vi "DSF.Engine.Memory.Cache.Plugin.Get Transfer Caches.vi"(8 "error in (no error)":errorcluster, 11 "Plugin Cache in":refnum<class "DSF.Engine.Memory.Cache.Plugin.lvclass">) -> (0 "error out":errorcluster, 2 "Transfer Caches":refnum<class "DSF.Engine.Memory.Cache.Transfer.lvclass">[](array[class]), 3 "Plugin Cache out":refnum<class "DSF.Engine.Memory.Cache.Plugin.lvclass">)   [LabVIEW 2016, in "DSF.Engine.lvlib" / "DSF.Engine.Memory.Cache.Plugin.lvclass"]
uses:
  DSF.Engine.Memory.Cache.Plugin.lvclass
  DSF.Engine.Memory.Cache.Transfer.lvclass
  DSF.Engine.Memory.Cache.Plugin.lvclass/DSF.Engine.Memory.Cache.Plugin.ctl
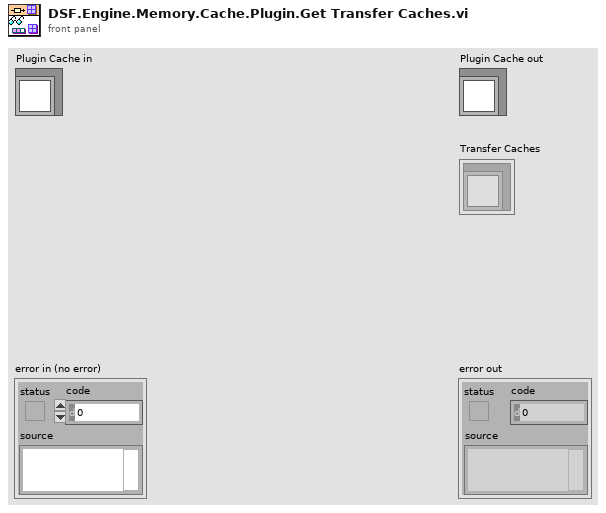
[diagram p1: front panel]
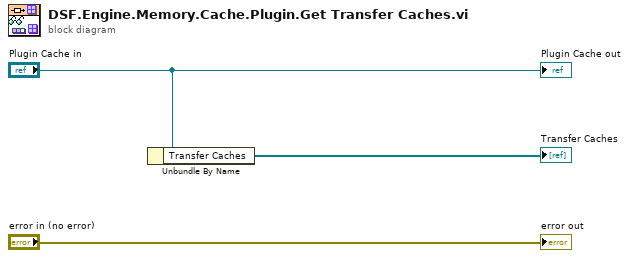
[diagram p0: block diagram]
diagram:
  n1 = Unbundle By Name("Plugin Cache in") -> ("Transfer Caches"=→"Transfer Caches":refnum<class "DSF.Engine.Memory.Cache.Transfer.lvclass">[])
  "error out" <- "error in (no error)"
  "Plugin Cache out" <- "Plugin Cache in"
